vi "Input.vi"(8 "error in (no error)":errorcluster, 11 "Pump Calibration Config in":T1={"Settings"={"Cycle Period"=500.0, "Ismatech"={"VISA resource name"="", "Simulated?"=TRUE, "Pump Number"=1.0, "Reverse?"=FALSE}, "Masterflex"={"VISA resource name"="", "Simulated?"=TRUE, "Pump Number"=1.0, "Reverse?"=FALSE}, "Bronkhorst M13 Flow Meter"={"VISA resource name"="", "Simulated?"=TRUE}, "PID 2 Parameters"={"Input Device"=enum."Default", "Output Device"=enum."Default"}, "Bronkhorst M14"={"VISA resource name"="", "Simulated?"=FALSE}, "Tacmina Settings"={"Analog DAQ Task"="", "Digital DAQ Task"=""}, "KNF SIMDOS Settings"={"VISA resource name"="", "Simulated?"=TRUE}, "VICI M50 Settings"={"VISA resource name"="", "Simulated?"=TRUE, "Pump Letter"="", "Reverse?"=FALSE}, "FLOM Settings"={"VISA resource name"="", "Simulated?"=TRUE, "Pump Number"=0.0}, "Calibration Limits"={"Minimum (ml/min)"=0.0, "Maximum (ml/min)"=0.0, "Steps"=0.0}, "SSI PR Settings"={"VISA resource name"="", "Simulated?"=FALSE}}, "Flowmeter Output"=0.0, "Density"=0.0, "FL Temp"=0.0, "Speed %"=0.0, "File Refnum"=refnum, "Pump On?"=enum."Not Initialized"} {"Settings"."Masterflex"."Pump Number" min=1.0 max=20.0 step=1.0; "Settings"."Ismatech"."Pump Number" min=1.0 max=20.0 step=1.0}) -> (0 "error out":errorcluster, 3 "Pump Calibration Config Out":T1={"Settings"={"Cycle Period"=500.0, "Ismatech"={"VISA resource name"="", "Simulated?"=TRUE, "Pump Number"=1.0, "Reverse?"=FALSE}, "Masterflex"={"VISA resource name"="", "Simulated?"=TRUE, "Pump Number"=1.0, "Reverse?"=FALSE}, "Bronkhorst M13 Flow Meter"={"VISA resource name"="", "Simulated?"=TRUE}, "PID 2 Parameters"={"Input Device"=enum."Default", "Output Device"=enum."Default"}, "Bronkhorst M14"={"VISA resource name"="", "Simulated?"=FALSE}, "Tacmina Settings"={"Analog DAQ Task"="", "Digital DAQ Task"=""}, "KNF SIMDOS Settings"={"VISA resource name"="", "Simulated?"=TRUE}, "VICI M50 Settings"={"VISA resource name"="", "Simulated?"=TRUE, "Pump Letter"="", "Reverse?"=FALSE}, "FLOM Settings"={"VISA resource name"="", "Simulated?"=TRUE, "Pump Number"=0.0}, "Calibration Limits"={"Minimum (ml/min)"=0.0, "Maximum (ml/min)"=0.0, "Steps"=0.0}, "SSI PR Settings"={"VISA resource name"="", "Simulated?"=FALSE}}, "Flowmeter Output"=0.0, "Density"=0.0, "FL Temp"=0.0, "Speed %"=0.0, "File Refnum"=refnum, "Pump On?"=enum."Not Initialized"} {"Settings"."Masterflex"."Pump Number" min=1.0 max=20.0 step=1.0; "Settings"."Ismatech"."Pump Number" min=1.0 max=20.0 step=1.0})   [LabVIEW 2018, in "Calibration.lvlib" / "Engine.lvlib"]
uses:
  Engine.lvlib
  Pump Calibration Config.ctl
  Pfizer Timed Seq/Software/Ismatec ISM 831C/Controls/Ismatech Settings Cluster.ctl
  Pfizer Timed Seq/Software/Masterflex 7550-30/Controls/Settings Cluster.ctl
  Pfizer Timed Seq/Software/Bronkhorst M13 Flow Meter/Settings Cluster.ctl
  Pfizer Timed Seq/Software/Measure Instrument/PID Input Enum.ctl
  Pfizer Timed Seq/Software/Measure Instrument/PID 2 Output Enum.ctl
  Pfizer Timed Seq/Software/Mettler Toledo/Controls/Settings Cluster.ctl
  Pfizer Timed Seq/Software/Tacmina QI/Tacmina QI DAQ Setting.ctl
  Pfizer Timed Seq/Software/KNF Pump/Settings Cluster plus SIMDOS.ctl
  Pfizer Timed Seq/Software/VICI M50 Party Mode/Settings Cluster.ctl
  Pfizer Timed Seq/Software/FLOM Pump/Settings Cluster.ctl
  Pfizer Timed Seq/Software/SSI PR Class/SSI PR Settings Cluster.ctl
  Pfizer Timed Seq/Software/Bronkhorst M13 Flow Meter/Bronkhorst M13 Flow Meter.lvlib
  Pfizer Timed Seq/Software/Bronkhorst M14 Flow Meter/Bronkhorst M14 Flow Meter.lvlib
  Pfizer Timed Seq/Software/VICI M50 Party Mode/VICI M6 M50 Party Mode.lvlib
  Pfizer Timed Seq/Software/Ismatec ISM 831C/Ismatec ISM 831C.lvlib
  Pfizer Timed Seq/Software/Masterflex 7550-30/Masterflex 7550-30.lvlib
  Pfizer Timed Seq/Software/Mettler Toledo/Mettler Toledo.lvlib
  Pfizer Timed Seq/Software/Tacmina QI/Tacmina QI.lvlib
  Pfizer Timed Seq/Software/KNF Pump/KNF SIMDOS.lvlib
  Pfizer Timed Seq/Software/FLOM Pump/FLOM Pump.lvlib
  Pfizer Timed Seq/Software/Calibration VIs/Calibration.lvlib
  Pfizer Timed Seq/Software/SSI PR Class/SSI PR Pump.lvlib
panel:
  # "Output Instruments"
  # "Input Instruments"
  # "Output Instruments"
  # "Input Instruments"
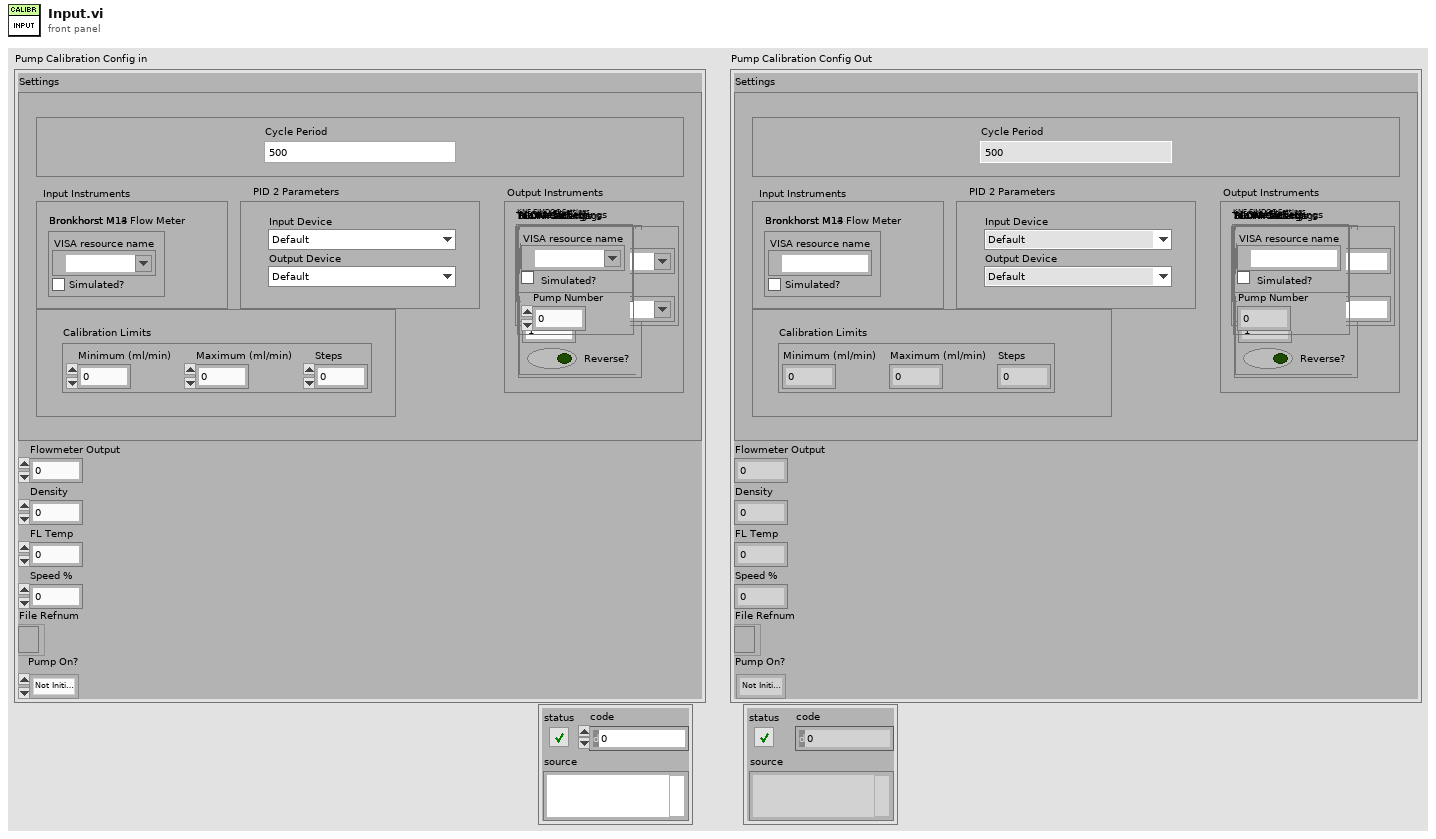
[diagram p1: front panel]
types:
  T1 = typedef "Calibration.lvlib/Pump Calibration Config.ctl" = cluster{"Settings":cluster{"Cycle Period":dbl, "Ismatech":T2, "Masterflex":T3, "Bronkhorst M13 Flow Meter":T4, "PID 2 Parameters":cluster{"Input Device":T5, "Output Device":T6}, "Bronkhorst M14":T7, "Tacmina Settings":T8, "KNF SIMDOS Settings":T9, "VICI M50 Settings":T10, "FLOM Settings":T11, "Calibration Limits":cluster{"Minimum (ml/min)":dbl, "Maximum (ml/min)":dbl, "Steps":dbl}, "SSI PR Settings":T12}, "Flowmeter Output":dbl, "Density":dbl, "FL Temp":dbl, "Speed %":dbl, "File Refnum":refnum<file>, "Pump On?":enum16{"Off", "On", "Not Initialized"}}
  T2 = typedef "Ismatec ISM 831C.lvlib/Ismatech Settings Cluster.ctl" = cluster{"VISA resource name":refnum<visa-resource-name>, "Simulated?":bool, "Pump Number":dbl, "Reverse?":bool}
  T3 = typedef "Masterflex 7550-30.lvlib/Settings Cluster.ctl" = cluster{"VISA resource name":refnum<visa-resource-name>, "Simulated?":bool, "Pump Number":dbl, "Reverse?":bool}
  T4 = typedef "Bronkhorst M13 Flow Meter.lvlib/Settings Cluster.ctl" = cluster{"VISA resource name":refnum<visa-resource-name>, "Simulated?":bool}
  T5 = typedef "PID Input Enum.ctl" = enum16{"Default", "Bronkhorst M13", "Bronkhorst M14", "Scale Rate of Change"}
  T6 = typedef "PID 2 Output Enum.ctl" = enum16{"Default", "Ismatec ISM 831C", "Masterflex 7550-30", "VICI", "Tacmina QI", "KNF SIMDOS", "ASIA Type C", "FLOM UI-22-11", "SSI PR"}
  T7 = typedef "Mettler Toledo.lvlib/Settings Cluster.ctl" = cluster{"VISA resource name":refnum<visa-resource-name>, "Simulated?":bool}
  T8 = typedef "Tacmina QI.lvlib/Tacmina QI DAQ Setting.ctl" = cluster{"Analog DAQ Task":refnum<k21>, "Digital DAQ Task":refnum<k21>}
  T9 = typedef "KNF SIMDOS.lvlib/Settings Cluster plus SIMDOS.ctl" = cluster{"VISA resource name":refnum<visa-resource-name>, "Simulated?":bool}
  T10 = typedef "VICI M6 M50 Party Mode.lvlib/Settings Cluster.ctl" = cluster{"VISA resource name":refnum<visa-resource-name>, "Simulated?":bool, "Pump Letter":string, "Reverse?":bool}
  T11 = typedef "FLOM Pump.lvlib/Settings Cluster.ctl" = cluster{"VISA resource name":refnum<visa-resource-name>, "Simulated?":bool, "Pump Number":dbl}
  T12 = typedef "SSI PR Pump.lvlib/SSI PR Settings Cluster.ctl" = cluster{"VISA resource name":refnum<visa-resource-name>, "Simulated?":bool}
  T13 = typedef "Bronkhorst M14 Flow Meter.lvlib/Settings Cluster.ctl" = cluster{"VISA resource name":refnum<visa-resource-name>, "Simulated?":bool}
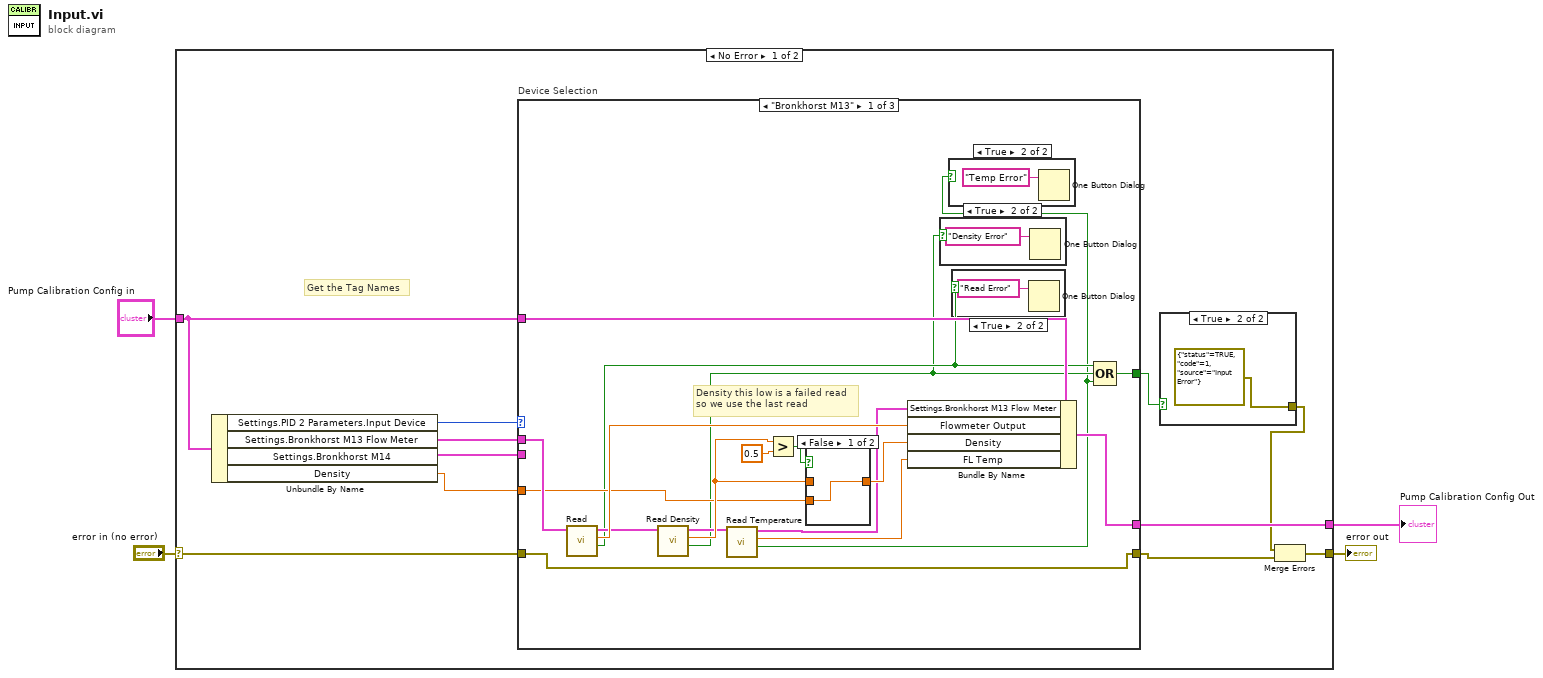
[diagram p0: block diagram]
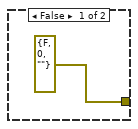
[diagram p2: hidden frame]
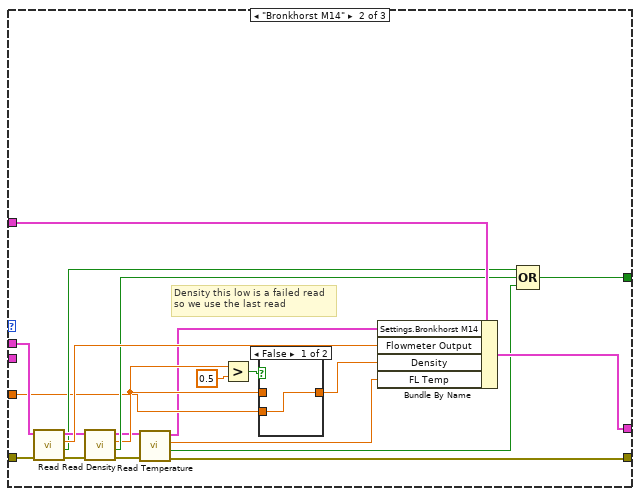
[diagram p7: hidden frame]
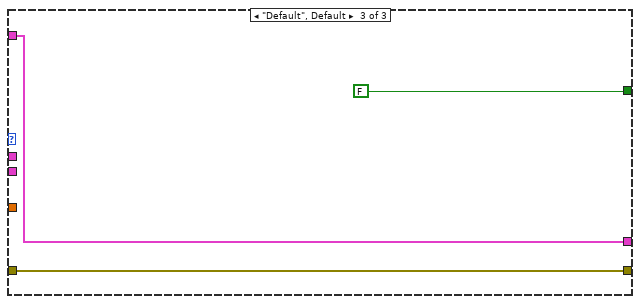
[diagram p9: hidden frame]
diagram:
  n1 = case shown="No Error" "error in (no error)" {
    selector: "error in (no error)" -> [w12 w68]
    tunnel: [w6 w68] -> w3
    tunnel: "Pump Calibration Config in" -> [w9 w67]
    tunnel: [w10 w67] -> w1
    frame No Error {
      # "Get the Tag Names"
      n2 = Unbundle By Name(w9) -> ("Settings.PID 2 Parameters.Input Device"=w15:T5, "Settings.Bronkhorst M13 Flow Meter"=w14:T4, "Settings.Bronkhorst M14"=w13:T7, "Density"=w11:dbl)
      n3 = case "Device Selection" shown="\"Bronkhorst M13\"" w15 {
        tunnel: w9 -> [w35 w61 w66]
        tunnel: [w34 w60 w66] -> w10
        tunnel: w14 -> [w32 w57 _]
        tunnel: w13 -> [_ _ _]
        tunnel: w12 -> [w21 w58 w65]
        tunnel: [w21 w43 w65] -> w8
        tunnel: [w30 w52 FALSE ("Connection Error")] -> w5
        tunnel: w11 -> [w25 w47 _]
        frame "Bronkhorst M13" {
          # "Density this low is a failed read\nso we use the last read"
          n4 = call "Read.vi"("Bronkhorst Settings in"=w32) -> ("Connection Error"=w20:bool, "flow"=w33:dbl, "Bronkhorst Settings out"=w31:T4)  [unwired: 7 in, 1 out]
          n5 = call "Read Density.vi"("Bronkhorst Settings in"=w31) -> ("Connection Error"=w19:bool, "Density kg/m^3"=w27:sgl, "Bronkhorst Settings out"=w24:T4)  [unwired: 7 in, 1 out]
          n6 = call "Read Temperature.vi"("Bronkhorst Settings in"=w24) -> ("Connection Error"=w18:bool, "Temp (C)"=w22:sgl, "Bronkhorst Settings out"=w23:T4)  [unwired: 7 in, 1 out]
          n7 = Greater?(x=w27, y=sgl 0.5) -> (0:w29:bool)
          n8 = case shown="False" w29 {
            tunnel: w27 -> [_ w40]
            tunnel: [w39 w40] -> w26
            tunnel: w25 -> [w39 _]
            frame False {
            }
            frame True {
            }
          }
          n9 = Bundle By Name(cluster=w35, "Settings.Bronkhorst M13 Flow Meter"=w23, "Flowmeter Output"=w33, "Density"=w26, "FL Temp"=w22) -> (w34:T1)
          n10 = case shown="True" w19 {
            frame False {
            }
            frame True {
              n11 = One Button Dialog(message="Density Error") -> ()  [unwired: 1 in, 1 out]
            }
          }
          n12 = case shown="True" w18 {
            frame False {
            }
            frame True {
              n13 = One Button Dialog(message="Temp Error") -> ()  [unwired: 1 in, 1 out]
            }
          }
          n14 = case shown="True" w20 {
            frame False {
            }
            frame True {
              n15 = One Button Dialog(message="Read Error") -> ()  [unwired: 1 in, 1 out]
            }
          }
          n16 = Compound Arithmetic op=OR(w20, w19, w18) -> (w30:bool)
        }
        frame "Bronkhorst M14" {
          # "Density this low is a failed read\nso we use the last read"
          n17 = call "Read.vi"("error in (no error)"=w58, "Bronkhorst Settings in"=w57) -> ("error out"=w56:errorcluster, "Connection Error"=w54:bool, "flow"=w59:dbl, "Bronkhorst Settings out"=w55:T13)  [unwired: 6 in]
          n18 = call "Read Density.vi"("error in (no error)"=w56, "Bronkhorst Settings in"=w55) -> ("error out"=w46:errorcluster, "Connection Error"=w53:bool, "Density kg/m^3"=w49:sgl, "Bronkhorst Settings out"=w45:T4)  [unwired: 6 in]
          n19 = call "Read Temperature.vi"("error in (no error)"=w46, "Bronkhorst Settings in"=w45) -> ("error out"=w43:errorcluster, "Connection Error"=w41:bool, "Temp (C)"=w42:sgl, "Bronkhorst Settings out"=w44:T4)  [unwired: 6 in]
          n20 = Greater?(x=w49, y=sgl 0.5) -> (0:w51:bool)
          n21 = case shown="False" w51 {
            tunnel: w49 -> [_ w63]
            tunnel: [w62 w63] -> w48
            tunnel: w47 -> [w62 _]
            frame False {
            }
            frame True {
            }
          }
          n22 = Bundle By Name(cluster=w61, "Settings.Bronkhorst M14"=w44, "Flowmeter Output"=w59, "Density"=w48, "FL Temp"=w42) -> (w60:T1)
          n23 = Compound Arithmetic op=OR(w54, w53, w41) -> (w52:bool)
        }
        frame "Default", Default {
        }
      }
      n24 = case shown="True" w5 {
        tunnel: [errorcluster {"status"=FALSE, "code"=0, "source"=""} ("error constant") errorcluster {"status"=TRUE, "code"=1, "source"="Input Error"} ("error constant")] -> w7
        frame False {
        }
        frame True {
        }
      }
      n25 = Merge Errors(w7, w8) -> (w6:errorcluster)
    }
    frame Error {
    }
  }
  "error out" <- w3
  "Pump Calibration Config Out" <- w1
